vi "XMLMetaDataToClusterOfArrays.vi"(8 "error in":errorcluster, 11 "XML File Path":path) -> (0 "error out":errorcluster, 1 "Number of Files Processed":i32, 3 "Results Cluster":T1)   [LabVIEW 2019, in "Analysis.lvlib"]
doc: "This VI converts Aquatrak calibration files in a base folder to a LabVIEW cluster of arrays. By converting the XML files to primative data types, analysis may be performed to analyze the efficiency, precision and accuracy of the calibrations."
uses:
  Analysis.lvlib
  <vilib>/Analysis/baseanly.llb/Mean (DBL).vi
  <vilib>/Utility/xml.llb/Read From XML File(string).vi
  <vilib>/Analysis/NI_AALBase.lvlib
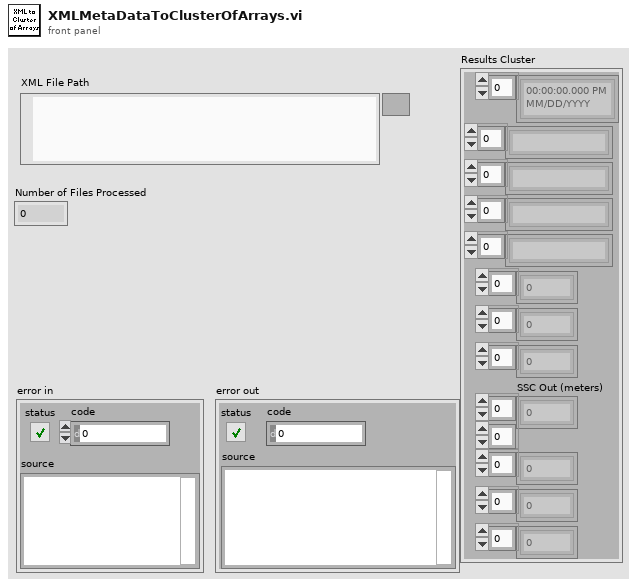
[diagram p1: front panel]
types:
  T1 = cluster{timestamp[], string[], string[], string[], string[], dbl[], dbl[], dbl[], "SSC Out (meters)":dbl[][], dbl[], dbl[], dbl[]}
  T2 = cluster{"date/time string":string, "Meta Data":cluster{"Calibration Location":string, "Operator Name":string, "Sensor SN":string, "Cal Tube SN":string, "Comments":string}, "Ring Time":dbl, "Error to Cal Hole (unused)":dbl, "Mean Offset":dbl, "Temp Out":dbl[], "Excitation Current":dbl, "SSC Out (meters)":dbl[], "Short Offset":dbl, "Mid Offset":dbl, "Long Offset":dbl}
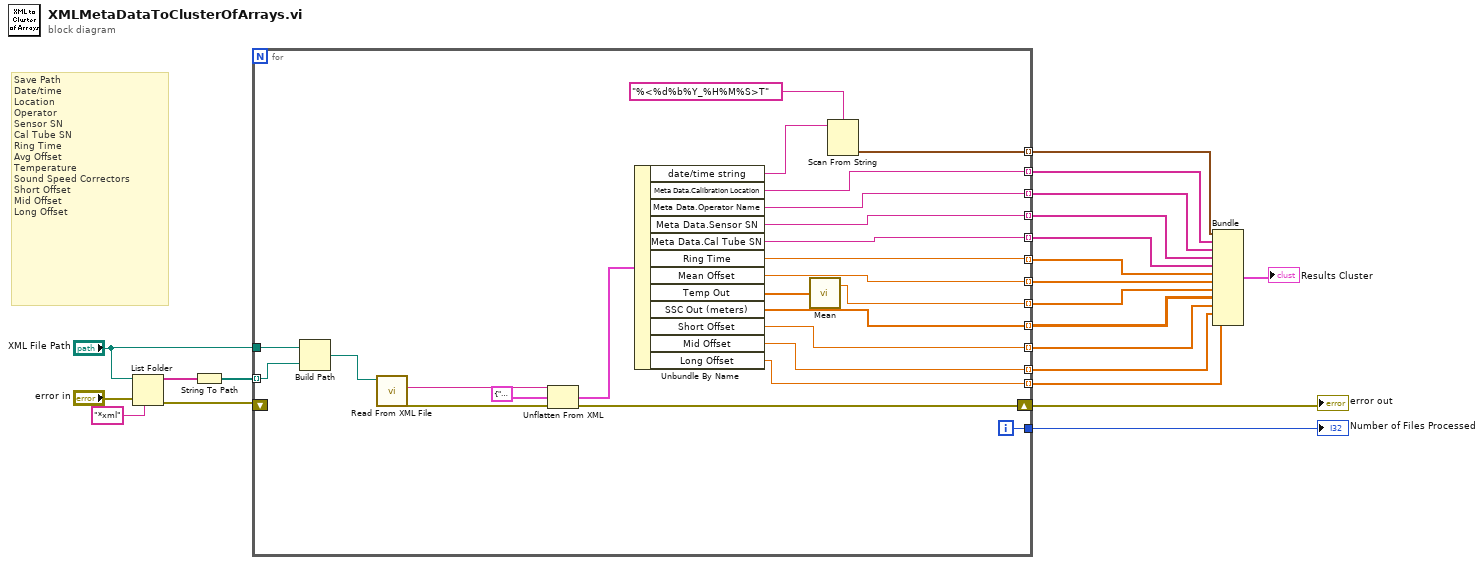
[diagram p0: block diagram]
diagram:
  # "Save Path\nDate/time\nLocation\nOperator\nSensor SN\nCal Tube SN\nRing Time\nAvg Offset\nTemperature\nSound Speed Correctors\nShort Offset\nMid Offset\nLong Offset"
  n1 = List Folder(path="XML File Path", pattern="*xml", error in="error in") -> (filenames=w21:string[], error out=w16:errorcluster)  [unwired: 1 in, 2 out]
  n2 = String To Path(string=w21) -> (path=w20:path[])
  n3 = for {
    tunnel: w20 -> [w42] mode=indexing
    tunnel: "XML File Path" -> [w43]
    tunnel: [w38] -> w15 mode=indexing
    tunnel: [w37] -> w14 mode=indexing
    tunnel: [w36] -> w13 mode=indexing
    tunnel: [w35] -> w12 mode=indexing
    tunnel: [w34] -> w4 mode=indexing
    tunnel: [w33] -> w11 mode=indexing
    tunnel: [w32] -> w10 mode=indexing
    tunnel: [w25] -> w9 mode=indexing
    tunnel: [w31] -> w8 mode=indexing
    tunnel: [w30] -> w7 mode=indexing
    tunnel: [w29] -> w6 mode=indexing
    shift-right: [w28] -> w18
    shift-left: w16 -> [_]
    tunnel: [w27] -> w5
    tunnel: [w24] -> w1 mode=indexing
    i -> [w27]
    n4 = Build Path(base path=w43, name or relative path=w42) -> (appended path=w41:path)
    n5 = call-poly <vilib>:"Read From XML File.vi"("XML File Path"=w41) -> ("error out"=w44:errorcluster, "XML Elements"=w45:string)  [unwired: 8 in, 1 out]
    n6 = Unflatten From XML(xml string=w45, type=T2 {"date/time string"="", "Meta Data"={"Calibration Location"="", "Operator Name"="", "Sensor SN"="", "Cal Tube SN"="", "Comments"=""}, "Ring Time"=0.0, "Error to Cal Hole (unused)"=0.0, "Mean Offset"=0.0, "Temp Out"=[], "Excitation Current"=0.0, "SSC Out (meters)"=[], "Short Offset"=0.0, "Mid Offset"=0.0, "Long Offset"=0.0} ("output cluster"), error in (no error)=w44) -> (value=w22:T2, error out=w28:errorcluster)
    n7 = Unbundle By Name(w22) -> ("date/time string"=w40:string, "Meta Data.Calibration Location"=w37:string, "Meta Data.Operator Name"=w36:string, "Meta Data.Sensor SN"=w35:string, "Meta Data.Cal Tube SN"=w34:string, "Ring Time"=w33:dbl, "Mean Offset"=w32:dbl, "Temp Out"=w26:dbl[], "SSC Out (meters)"=w31:dbl[], "Short Offset"=w30:dbl, "Mid Offset"=w29:dbl, "Long Offset"=w24:dbl)
    n8 = call-poly <vilib>:"Mean.vi"("X"=w26) -> ("mean"=w25:dbl)  [unwired: 1 out]
    n9 = Scan From String(format string="%<%d%b%Y_%H%M%S>T" ("time format string (%c)"), input string=w40) -> (output 1=w38:timestamp)  [unwired: 3 in, 3 out]
  }
  "error out" <- w18
  "Number of Files Processed" <- w5
  n10 = Bundle(w15, w14, w13, w12, w4, w11, w10, w9, "SSC Out (meters)"=w8, w7, w6, w1) -> (→"Results Cluster":T1)  [unwired: 1 in]
